vi "Assignment 3.vi"() -> ()   [LabVIEW 2021]
panel:
  out "Warranty":dbl
  out "Power":dbl
  out "Price":dbl
  in  "Product":u16(ring) items=["Samsung", "LG", "Bosch"]
  in  "stop":bool
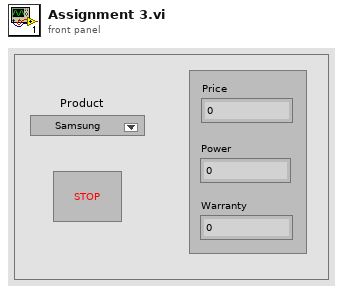
[diagram p1: front panel]
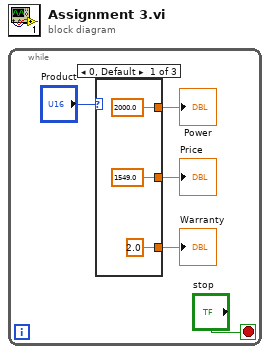
[diagram p0: block diagram]
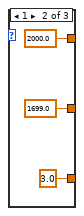
[diagram p2: hidden frame]
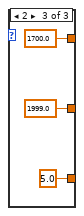
[diagram p3: hidden frame]
diagram:
  n1 = while {
    stop <- "stop" stop-if-true
    n2 = case shown="0, Default" "Product" {
      tunnel: [1549.0 1699.0 1999.0] -> w3
      tunnel: [2000.0 2000.0 1700.0] -> w2
      tunnel: [2.0 3.0 5.0] -> w1
      frame 0, Default {
      }
      frame 1 {
      }
      frame 2 {
      }
    }
    "Price" <- w3
    "Power" <- w2
    "Warranty" <- w1
  }
